vi "Auto settings.vi"(8 "error in (no error)":errorcluster, 10 "Array":dbl[](array[numeric]), 11 "Fixture in":refnum<class "Fixture.lvclass">) -> (0 "error out":errorcluster, 3 "Fixture out":refnum<class "Fixture.lvclass">)   [LabVIEW 2018, in "Fixture.lvclass"]
uses:
  Fixture.lvclass
  Fixture.lvclass/Fixture.ctl
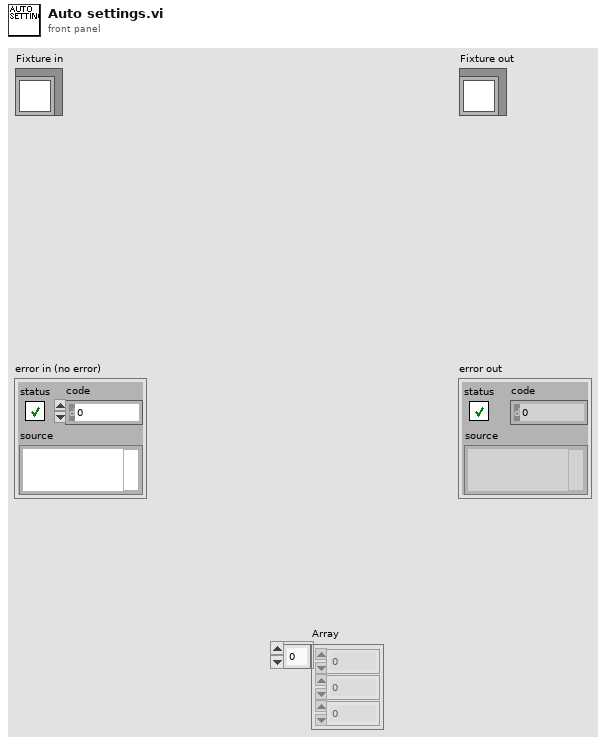
[diagram p1: front panel]
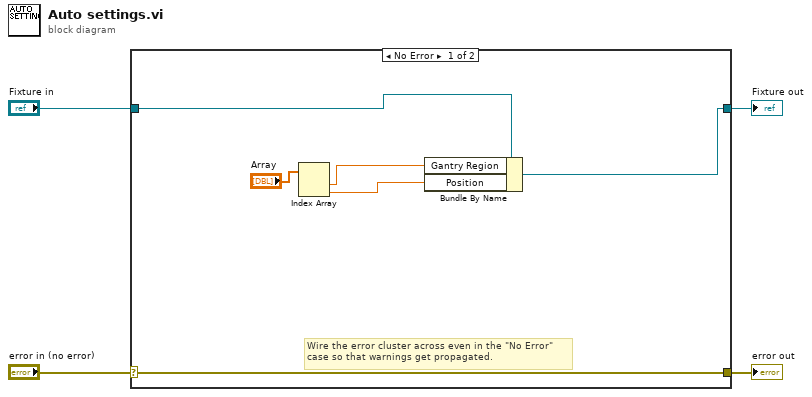
[diagram p0: block diagram]
diagram:
  n1 = case shown="No Error" "error in (no error)" {
    selector: "error in (no error)" -> [w10 w12]
    tunnel: [w10 w12] -> w3
    tunnel: [w8 w11] -> w1
    tunnel: "Fixture in" -> [w9 w11]
    frame No Error {
      # "Wire the error cluster across even in the \"No Error\"\ncase so that warnings get propagated."
      n2 = Index Array(array="Array") -> (element #1=w6:dbl, element #2=w5:dbl)  [unwired: 2 in]
      n3 = Bundle By Name(cluster=w9, "Gantry Region"=w6, "Position"=w5) -> (w8:refnum<class "Fixture.lvclass">)
    }
    frame Error {
    }
  }
  "error out" <- w3
  "Fixture out" <- w1
